vi "Inst.AH2500.GetPublicEvents.vi"(8 "error in (no error)":errorcluster, 11 "Inst.AH2500 in":refnum<class "Inst.AH2500.lvclass">) -> (0 "error out":errorcluster, 2 "Inst.AH2500 Public Events":T1, 3 "Inst.AH2500 out":refnum<class "Inst.AH2500.lvclass">)   [LabVIEW 2019, in "Inst.AH2500.lvclass"]
uses:
  Inst.AH2500.lvclass
  Typedefs/PublicEvents--Cluster.ctl
  Typedefs/PublicEvents--Inst.AH2500.MessageFromProcess.ctl
  <userlib>/LevyLab/RemoteControl/RemoteControl/Typedefs/Message--Cluster.ctl
  Inst.AH2500.lvclass/Inst.AH2500.ctl
  <userlib>/LevyLab/RemoteControl/RemoteControl/RemoteControl.lvclass
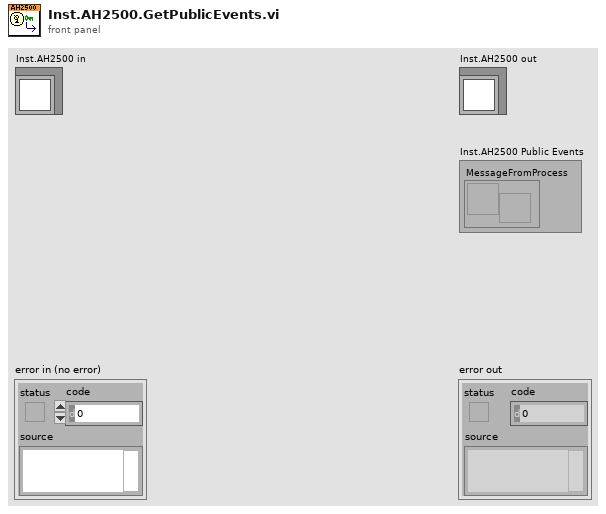
[diagram p1: front panel]
types:
  T1 = typedef "Inst.AH2500.lvclass/PublicEvents--Cluster.ctl" = cluster{"MessageFromProcess":refnum<user-event>}
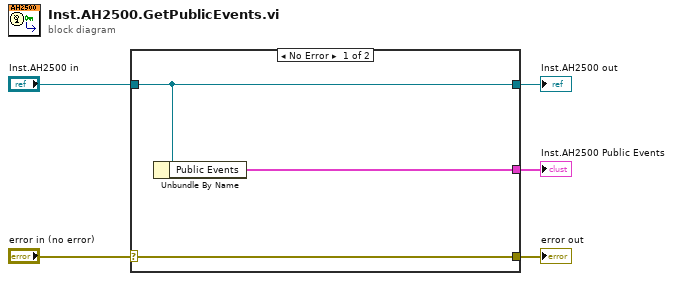
[diagram p0: block diagram]
diagram:
  n1 = case shown="No Error" "error in (no error)" {
    selector: "error in (no error)" -> [w8 w9]
    tunnel: [w8 w9] -> w4
    tunnel: [w7 w10] -> w2
    tunnel: "Inst.AH2500 in" -> [w7 w10]
    tunnel: [w6 _] -> w1
    frame No Error {
      n2 = Unbundle By Name(w7) -> ("Public Events"=w6:T1)
    }
    frame Error {
    }
  }
  "error out" <- w4
  "Inst.AH2500 out" <- w2
  "Inst.AH2500 Public Events" <- w1
